vi "niDTS GNSS GPS Rx RF Test Initialize.vi"(0 "Dut Reference":T2, 5 "SystemTechnologyCatalog":refnum<class "niDTS SystemTechnologyCatalog.lvclass">, 7 "SystemDut":refnum<class "niDTS SystemDut.lvclass">, 9 "Logger Reference":T1, 11 "error in (no error)":errorcluster) -> (4 "Dummy Test Handle out":T3, 6 "AllowAsync":bool=TRUE, 15 "error out":errorcluster)   [LabVIEW 2014, in "niDTS GNSS.lvlib"]
uses:
  niDTS GNSS.lvlib
  RF Test/Includes/niDTS GNSS RF Test INC Handle.ctl
  RF Test/Objects/BASE_class/niDTS GNSS RF Test.lvclass
  Framework/Dut/Includes/niDTS Dut INC Handle.ctl
  Framework/Dut/Objects/BASE_class/niDTS Dut.lvclass
  Framework/Logger/Includes/niDTS Logger INC Handle.ctl
  Framework/Logger/Objects/BASE_class/niDTS Logger.lvclass
  TestStand/Station/Objects/SystemTechnologyCatalog/niDTS SystemTechnologyCatalog.lvclass
  TestStand/Station/Objects/SystemDut/niDTS SystemDut.lvclass
  TestStand/niDTS TestStand.lvlib
  Framework/niDTS Framework.lvlib
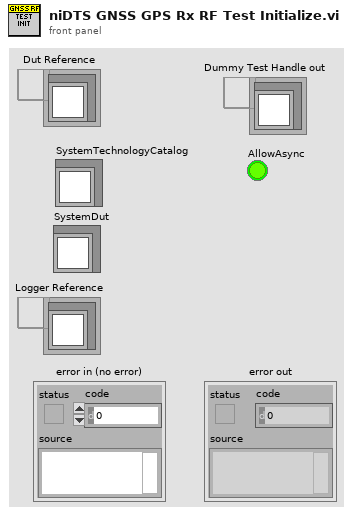
[diagram p1: front panel]
types:
  T1 = typedef "niDTS Framework.lvlib/niDTS Logger INC Handle.ctl" = refnum<data-value>
  T2 = typedef "niDTS Framework.lvlib/niDTS Dut INC Handle.ctl" = refnum<data-value>
  T3 = typedef "niDTS GNSS.lvlib/niDTS GNSS RF Test INC Handle.ctl" = refnum<data-value>
  T4 = typedef "niDTS TestStand.lvlib/niDTS TestStep INC Handle.ctl" = refnum<data-value>
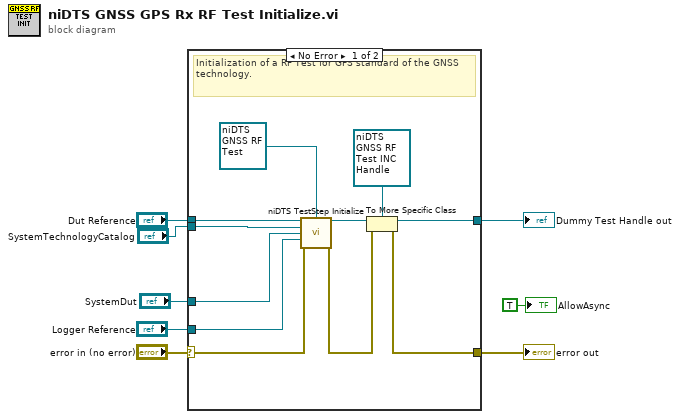
[diagram p0: block diagram]
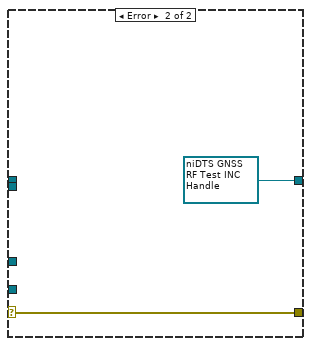
[diagram p2: hidden frame]
diagram:
  n1 = case shown="No Error" "error in (no error)" {
    selector: "error in (no error)" -> [w11 w21]
    tunnel: "Dut Reference" -> [w19 _]
    tunnel: [w10 T3 refnum ("Template Tx Test Handle")] -> w7
    tunnel: [w9 w21] -> w6
    tunnel: "Logger Reference" -> [w16 _]
    tunnel: "SystemTechnologyCatalog" -> [w13 _]
    tunnel: "SystemDut" -> [w12 _]
    frame No Error {
      # "Initialization of a RF Test for GPS standard of the GNSS \ntechnology."
      n2 = call "niDTS TestStep Initialize.vi"("Dut Handle"=w19, "Test Type"=refnum<class "niDTS GNSS RF Test.lvclass"> refnum ("Dummy Test.lvlib:Dummy Test.lvclass"), "SystemTechnologyCatalog"=w13, "SystemDut"=w12, "Logger Reference"=w16, "error in (no error)"=w11) -> ("Test Handle out"=w18:T4, "error out"=w17:errorcluster)  [unwired: 8 in]
      n3 = To More Specific Class(target class=T3 refnum ("Template Tx Test Handle"), reference=w18, error in=w17) -> (specific class reference=w10:T3, error out=w9:errorcluster)
    }
    frame Error {
    }
  }
  "error out" <- w6
  "Dummy Test Handle out" <- w7
  "AllowAsync" <- TRUE ("AllowAsync")
